vi "Initialize_Paths-2.vi"(4 "Test or Processing?":bool, 5 "start path":path, 6 "AVI File Path #2":path, 7 "AVI File Path #1":path) -> (0 "ERROR OUT":errorcluster, 1 "TI":dbl, 2 "AVI File Path #2 OUT":path, 3 "AVI File Path #1 OUT":path)   [LabVIEW 2017]
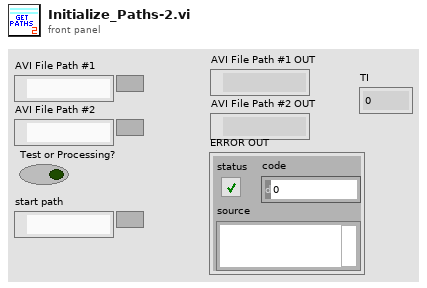
[diagram p1: front panel]
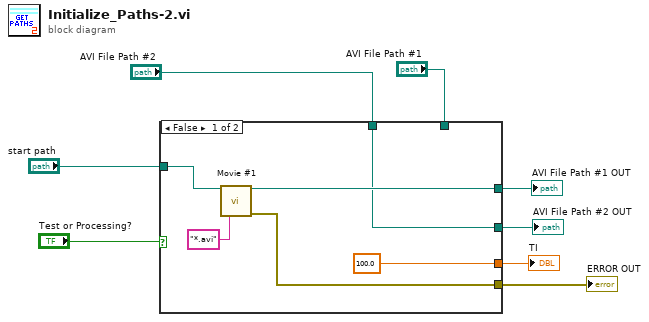
[diagram p0: block diagram]
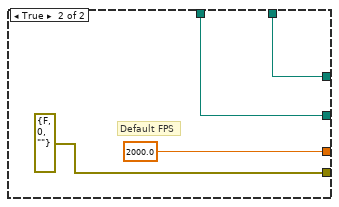
[diagram p2: hidden frame]
diagram:
  n1 = case shown="False" "Test or Processing?" {
    tunnel: [w13 w17] -> w5
    tunnel: [w9 w16] -> w4
    tunnel: [w11 errorcluster {"status"=FALSE, "code"=0, "source"=""} ("error out")] -> w3
    tunnel: [100.0 ("TI") 2000.0 ("TI")] -> w2
    tunnel: "AVI File Path #1" -> [_ w17]
    tunnel: "AVI File Path #2" -> [w9 w16]
    tunnel: "start path" -> [w12 _]
    frame False {
      n2 = call "Movie #1"("start path"=w12, "pattern (all files)"="*.avi") -> ("selected path"=w13:path, "error out"=w11:errorcluster)  [unwired: 10 in, 2 out]
    }
    frame True {
      # "Default FPS"
    }
  }
  "AVI File Path #1 OUT" <- w5
  "AVI File Path #2 OUT" <- w4
  "ERROR OUT" <- w3
  "TI" <- w2
